vi "get exposure time.vi"(8 "error in (no error)":errorcluster, 11 "Thorcam in":refnum<class "Thorcam.lvclass">) -> (0 "error out":errorcluster, 1 "exposure time":dbl[unit], 3 "Thorcam out":refnum<class "Thorcam.lvclass">)   [LabVIEW 2012, in "Thorcam.lvclass"]
uses:
  Thorcam.lvclass
  Thorcam.lvclass/Thorcam.ctl
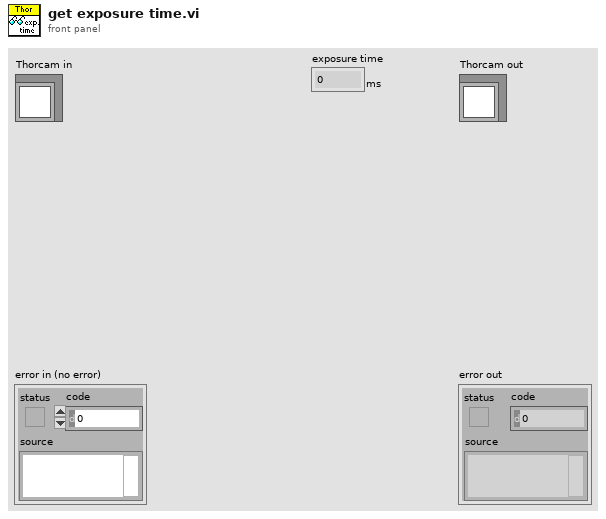
[diagram p1: front panel]
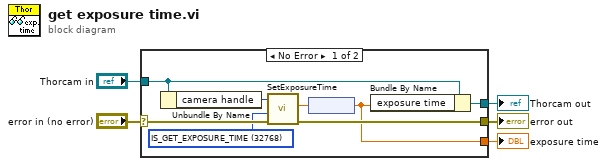
[diagram p0: block diagram]
diagram:
  n1 = case shown="No Error" "error in (no error)" {
    selector: "error in (no error)" -> [w12 w15]
    tunnel: [w11 w15] -> w4
    tunnel: [w8 w14] -> w2
    tunnel: "Thorcam in" -> [w9 w14]
    tunnel: [w6 _] -> w1
    frame No Error {
      w10 = u16 32768 items=["IS_SET_EXPOSURE_TIME"=32900, "IS_GET_EXPOSURE_TIME"=32768, "IS_GET_DEFAULT_EXPOSURE"=32769] ("Mode")
      n2 = Unbundle By Name(w9) -> ("camera handle"=w13:u32)
      n3 = call <instrlib>:"SetExposureTime.vi"("error in"=w12, "Mode"=w10, "Camera Handle In"=w13) -> ("error out"=w11:errorcluster, "new exposure time"=w7:dbl)  [unwired: 6 in, 1 out]
      n4 = node(w7) -> (w6:dbl[unit])
      n5 = Bundle By Name(cluster=w9, "exposure time"=w6) -> (w8:refnum<class "Thorcam.lvclass">)
    }
    frame Error {
    }
  }
  "error out" <- w4
  "Thorcam out" <- w2
  "exposure time" <- w1
